vi "MapDrop.vi"(1 "Name":string, 2 "Map In":variant) -> (0 "Map Out":variant)   [LabVIEW 2011]
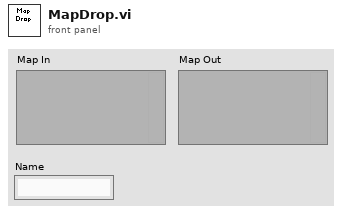
[diagram p1: front panel]
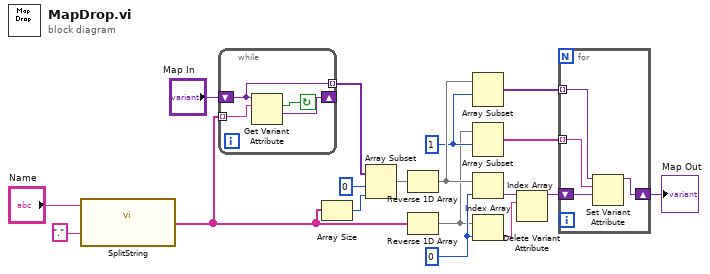
[diagram p0: block diagram]
diagram:
  w3 = 1 ("index")
  w8 = 0 ("index")
  n1 = call "SplitString.vi"("Delimeter"=".", "Name"="Name") -> ("Array"=w13:string[])
  n2 = while {
    tunnel: w13 -> [w22] mode=indexing
    shift-right: [w21] -> _
    shift-left: "Map In" -> [w19]
    tunnel: [w19] -> w14 mode=indexing
    stop <- w20 continue-if-true
    n3 = Get Variant Attribute(Variant=w19, name=w22) -> (found=w20:bool, value=w21:variant)  [unwired: 2 in, 2 out]
  }
  n4 = Array Size(array=w13) -> (size(s)=w12:i32)
  n5 = Array Subset(array=w14, index=0, length=w12) -> (w10:variant[])
  n6 = Reverse 1D Array(array=w10) -> (reversed array=w5:variant[])
  n7 = Reverse 1D Array(array=w13) -> (reversed array=w2:string[])
  n8 = Array Subset(array=w5, index=w3) -> (w4:variant[])  [unwired: 1 in]
  n9 = Array Subset(array=w2, index=w3) -> (w1:string[])  [unwired: 1 in]
  n10 = Index Array(array=w5, index=w8) -> (element=w9:variant)
  n11 = Index Array(array=w2, index=w8) -> (element=w7:string)
  n12 = Delete Variant Attribute(6:w7, 7:w9) -> (3:w6:variant)  [unwired: 1 in, 2 out]
  n13 = for {
    tunnel: w1 -> [w25] mode=indexing
    tunnel: w4 -> [w26] mode=indexing
    shift-right: [w23] -> w15
    shift-left: w6 -> [w24]
    n14 = Set Variant Attribute(Variant=w26, name=w25, value=w24) -> (Variant out=w23:variant)  [unwired: 1 in, 2 out]
  }
  "Map Out" <- w15
